vi "Scan Engine Update RemIO Subpanel.vi"(7 "SubPanel Event":refnum<user-event>, 8 "error in (no error)":errorcluster, 9 "SubPanel Ref":refnum<vi>, 10 "RemIO Module In":refnum<class "RemIO Module.lvclass">, 11 "Node Ptr In":T1 format="%.0x") -> (0 "error out":errorcluster, 2 "RemIO Module Out":refnum<class "RemIO Module.lvclass">, 3 "Node Ptr Out":T1 format="%.0x")   [LabVIEW 2019, in "SEECD System Explorer.lvlib"]
uses:
  SEECD System Explorer.lvlib
  <vilib>/NI VeriStand/Custom Device API/Custom Device Item Ref.ctl
  Modules.lvlibp/RSI Module/SubPanel Command.ctl
  Modules.lvlibp/RemIO Module/RemIO Module.lvclass
  <vilib>/Utility/miscctls.llb/LVRectTypeDef.ctl
  Shared/Globals/SubPanel Controls.vi
  Shared/SEECD Shared.lvlib
  <vilib>/NI VeriStand/Custom Device API/Custom Device API.lvlib
  Modules.lvlibp/RSI Module/RSI Module.lvclass
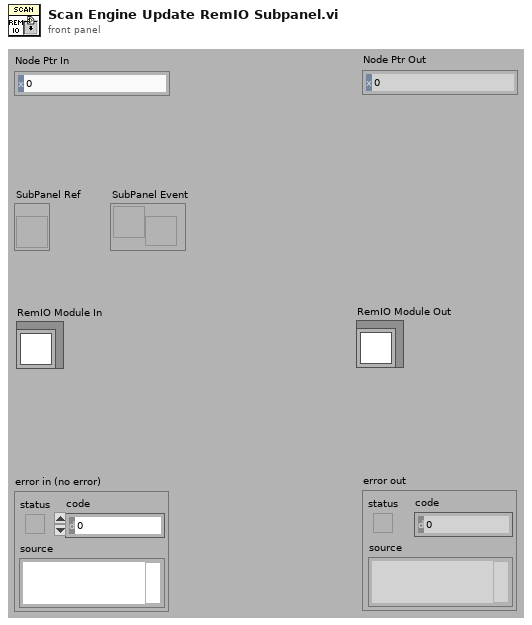
[diagram p1: front panel]
types:
  T1 = typedef "Custom Device API.lvlib/Custom Device Item Ref.ctl" = u64
  T2 = typedef "LVRectTypeDef.ctl" = cluster{"Left":i16, "Top":i16, "Right":i16, "Bottom":i16}
  T3 = typedef "LVBoundsTypeDef.ctl" = cluster{"Width":u32, "Height":u32}
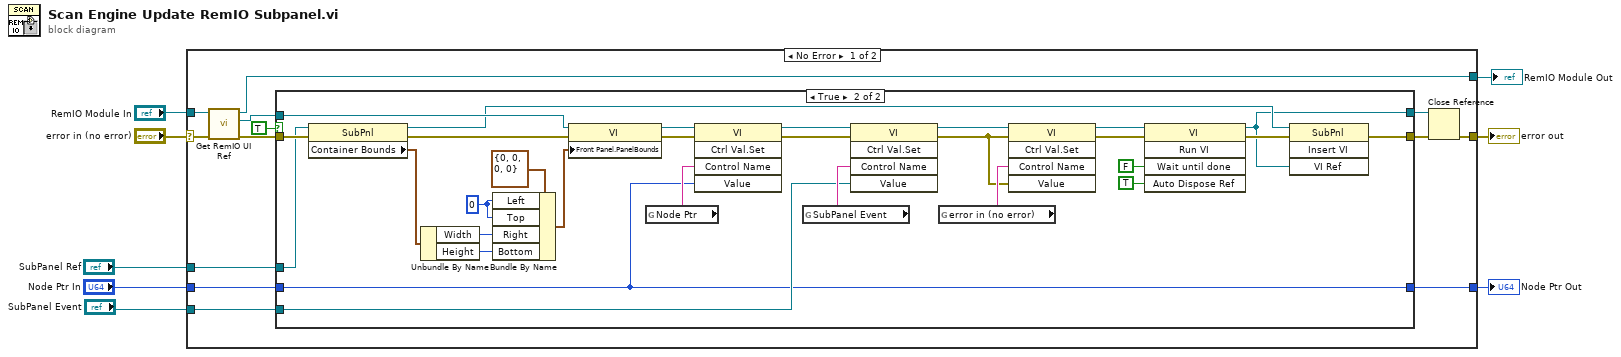
[diagram p0: block diagram]
diagram:
  n1 = case shown="No Error" "error in (no error)" {
    selector: "error in (no error)" -> [w13 w56]
    tunnel: "SubPanel Ref" -> [w21 _]
    tunnel: [w18 w56] -> w7
    tunnel: "Node Ptr In" -> [w17 w55]
    tunnel: "SubPanel Event" -> [w16 _]
    tunnel: "RemIO Module In" -> [w14 w54]
    tunnel: [w9 w54] -> w1
    tunnel: [w15 w55] -> w4
    frame No Error {
      n2 = call-dynamic "Get RemIO UI Ref.vi"("error in (no error)"=w13, "RemIO Module in"=w14) -> ("error out"=w12:errorcluster, "VI Refnum"=w11:refnum<vi>, "RemIO Module out"=w9:refnum<class "RemIO Module.lvclass">)  [unwired: 7 in]
      n3 = case shown="True" TRUE {
        tunnel: w21 -> [_ w31]
        tunnel: w11 -> [w23 w48]
        tunnel: [w23 w25] -> w20
        tunnel: [w24 w26] -> w19
        tunnel: w17 -> [w22 w32]
        tunnel: w12 -> [w24 w36]
        tunnel: w16 -> [_ w33]
        tunnel: [w22 w32] -> w15
        frame False {
        }
        frame True {
          w51 = i16 0 ("Left")
          n4 = property class="SubPnl"(reference=w31, error in=w36) -> (reference out=w28:refnum<vi>, error out=w35:errorcluster, "Container Bounds"=w49:T3)
          n5 = Unbundle By Name(w49) -> ("Width"=w52:u32, "Height"=w53:u32)
          n6 = Bundle By Name(cluster=T2 {"Left"=0, "Top"=0, "Right"=0, "Bottom"=0} ("Front Panel Window:Panel Bounds"), "Left"=w51, "Top"=w51, "Right"=w52, "Bottom"=w53) -> (w47:T2)
          n7 = property class="VI"(reference=w48, error in=w35, "Front Panel.PanelBounds"=w47) -> (reference out=w46:refnum<vi>, error out=w45:errorcluster)
          n8 = global read "SubPanel Controls.vi" "Node Ptr"() -> (w37:string)
          n9 = invoke class="VI" method="Ctrl Val.Set"(reference=w46, error in=w45, "Control Name"=w37, "Value"=w32) -> (reference out=w44:refnum<vi>, error out=w43:errorcluster)  [unwired: 1 in, 3 out]
          n10 = global read "SubPanel Controls.vi" "SubPanel Event"() -> (w34:string)
          n11 = invoke class="VI" method="Ctrl Val.Set"(reference=w44, error in=w43, "Control Name"=w34, "Value"=w33) -> (reference out=w30:refnum<vi>, error out=w29:errorcluster)  [unwired: 1 in, 3 out]
          n12 = global read "SubPanel Controls.vi" "error in (no error)"() -> (w38:string)
          n13 = invoke class="VI" method="Ctrl Val.Set"(reference=w30, error in=w29, "Control Name"=w38, "Value"=w29) -> (reference out=w42:refnum<vi>, error out=w41:errorcluster)  [unwired: 1 in, 3 out]
          n14 = invoke class="VI" method="Run VI"(reference=w42, error in=w41, "Wait until done"=FALSE ("Wait Until Done"), "Auto Dispose Ref"=TRUE ("Auto Dispose Reference")) -> (reference out=w25:refnum<vi>, error out=w27:errorcluster)  [unwired: 1 in, 3 out]
          n15 = invoke class="SubPnl" method="Insert VI"(reference=w28, error in=w27, "VI Ref"=w25) -> (error out=w26:errorcluster)  [unwired: 1 in, 3 out]
        }
      }
      n16 = Close Reference(reference=w20, error in (no error)=w19) -> (error out=w18:errorcluster)
    }
    frame Error {
    }
  }
  "error out" <- w7
  "Node Ptr Out" <- w4
  "RemIO Module Out" <- w1
